vi "InterpretSignal.vi"(1 "String in":string) -> (0 "String out":string)   [LabVIEW 2016]
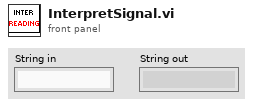
[diagram p1: front panel]
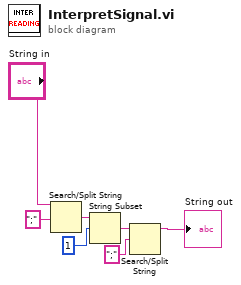
[diagram p0: block diagram]
diagram:
  n1 = Search/Split String(string="String in", search string/char (-)=";") -> (match + rest of string=w5:string)  [unwired: 1 in, 2 out]
  n2 = String Subset(string=w5, offset (0)=1) -> (substring=w3:string)  [unwired: 1 in]
  n3 = Search/Split String(string=w3, search string/char (-)=";") -> (substring before match=→"String out":string)  [unwired: 1 in, 2 out]
